vi "HGCalSensorTestingPanel.vi"() -> ()   [LabVIEW 2015]
uses:
  <vilib>/Utility/file.llb/Write Delimited Spreadsheet (string).vi
panel:
  out "XY Graph 2":cluster{"Y":dbl[], "Y":dbl[]}[](graph)
  out "return count 5":u32
  in  "write buffer 2":string
  out "return count 4":u32
  in  "VISA QT7600":refnum<visa-resource-name>
  in  "write buffer":string
  out "VISA out 3":refnum<visa-resource-name>
  out "return count 3":u32
  in  "byte count 2":u32
  out "XY Graph":cluster{"Y":dbl[], "Y":dbl[]}[](graph)
  out "VISA out 2":refnum<visa-resource-name>
  out "return count 2":u32
  out "error out 2":errorcluster
  in  "byte count":u32
  in  "HP":refnum<visa-resource-name>
  out "VISA out":refnum<visa-resource-name>
  out "return count":u32
  in  "error in":errorcluster
  in  "Switch":refnum<visa-resource-name>
  in  "Measurement Data":string[][](table)
  in  "OK Button":bool
  in  "Delay (s):":dbl
  in  "Channel:":dbl
  in  "Voltage (V):":dbl
  out "Channel:":dbl format="%#3_6g"
  out "mV(nA)":dbl
  out "pF":dbl
  out "V":dbl
  out "nA":dbl
  # "C"
  # "A"
  # "V"
  # "1M"
  # "1M"
  # "Single Measurement"
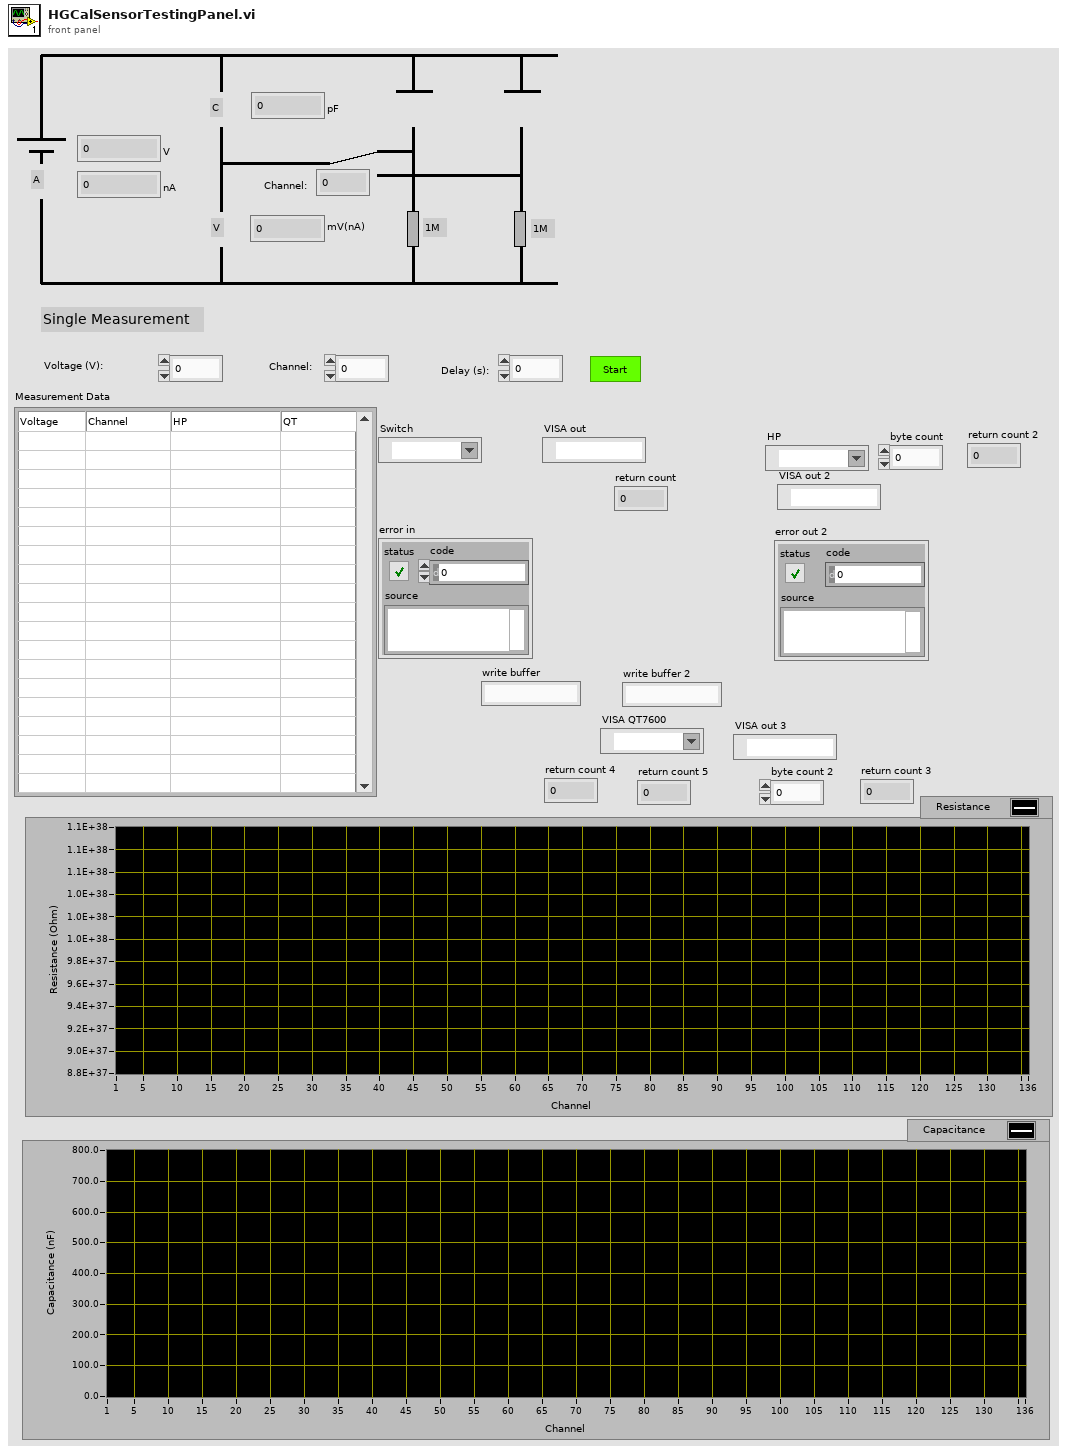
[diagram p1: front panel]
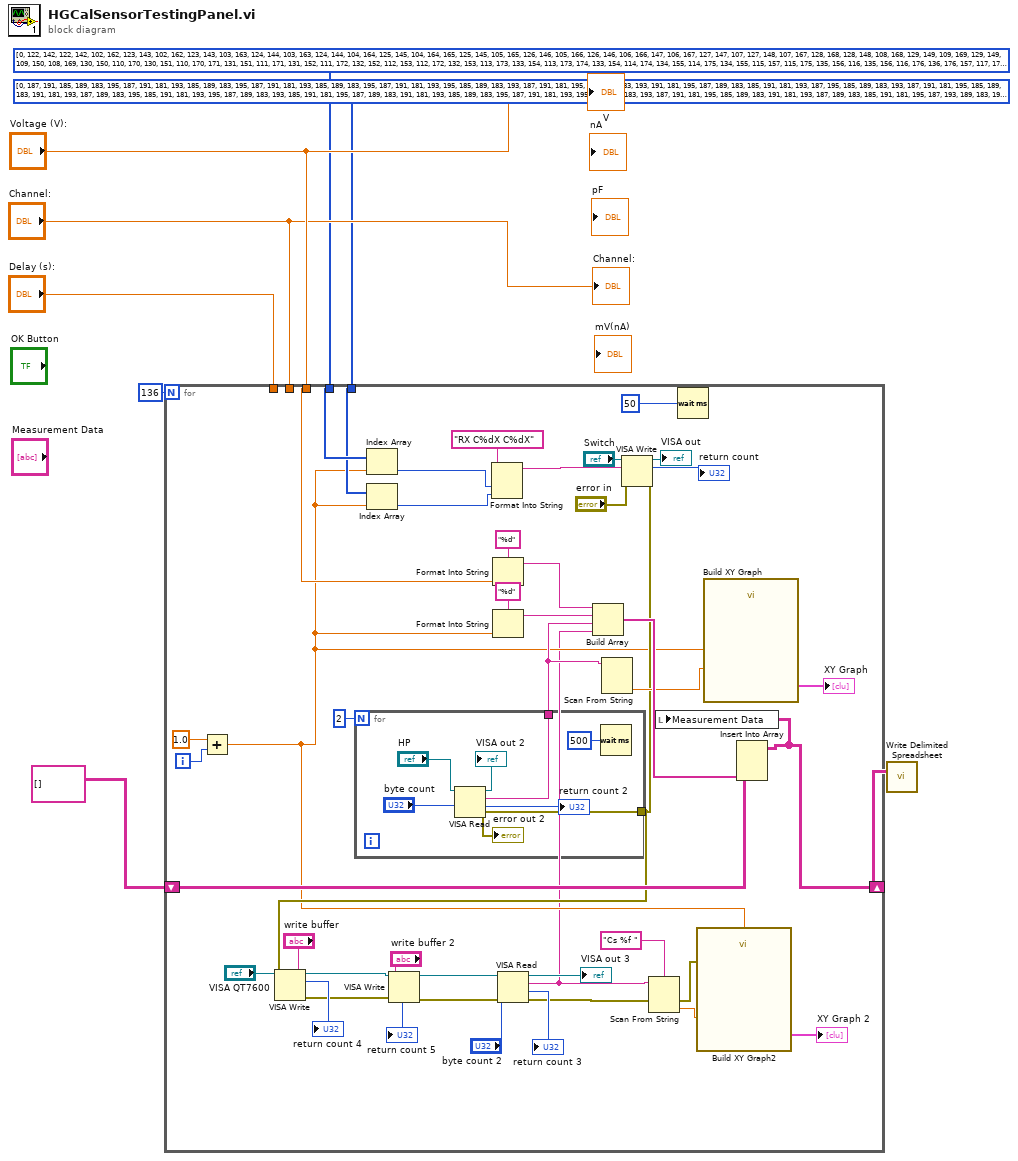
[diagram p0: block diagram]
diagram:
  n1 = for {
    N: 136 -> [_]
    shift-right: [w44] -> w3
    shift-left: string[][] [] -> [w53]
    tunnel: "Voltage (V):" -> [w52]
    tunnel: "Channel:" -> [_]
    tunnel: "Delay (s):" -> [_]
    tunnel: i32[] [0, 122, 142, 122, 142, 102, 162, 123, 143, 102, 162, 123, 143, 103, 163, 124, 144, 103, 163, 124, 144, 104, 164, 125, 145, 104, 164, 165, 125, 145, 105, 165, 126, 146, 105, 166, 126, 146, 106, 166, 147, 106, 167, 127, 147, 107, 127, 148, 107, 167, 128, 168, 128, 148, 108, 168, 129, 149, 109, 169, 129, 149, 109, 150, 108, 169, 130, 150, 110, 170, 130, 151, 110, 170, 171, 131, 151, 111, 171, 131, 152, 111, 172, 132, 152, 112, 153, 112, 172, 132, 153, 113, 173, 133, 154, 113, 173, 174, 133, 154, 114, 174, 134, 155, 114, 175, 134, 155, 115, 157, 115, 175, 135, 156, 116, 135, 156, 116, 176, 136, 176, 157, 117, 177, 136, 158, 117, 177, 137, 137, 158, 118, 178, 138, 138, 159, 178] -> [w43]
    tunnel: i32[] [0, 187, 191, 185, 189, 183, 195, 187, 191, 181, 193, 185, 189, 183, 195, 187, 191, 181, 193, 185, 189, 183, 195, 187, 191, 181, 193, 195, 185, 189, 183, 193, 187, 191, 181, 195, 185, 189, 183, 193, 191, 181, 195, 187, 189, 183, 185, 191, 181, 193, 187, 195, 185, 189, 183, 193, 187, 191, 181, 195, 185, 189, 183, 191, 181, 193, 187, 189, 183, 195, 185, 191, 181, 193, 195, 187, 189, 183, 193, 185, 191, 181, 195, 187, 189, 183, 191, 181, 193, 185, 189, 183, 195, 187, 191, 181, 193, 195, 185, 189, 183, 193, 187, 191, 181, 195, 185, 189, 183, 191, 181, 193, 187, 189, 183, 185, 191, 181, 195, 187, 193, 189, 183, 195, 185, 191, 181, 193, 187, 185, 189, 183, 195, 187, 185, 191, 193] -> [w42]
    i -> [w46]
    n2 = Add(x=1.0, y=w46) -> (x+y=w14:dbl)
    n3 = Index Array(array=w43, index=w14) -> (element=w41:i32)
    n4 = Index Array(array=w42, index=w14) -> (element=w40:i32)
    n5 = Format Into String(format string="RX C%dX C%dX", w41, w40) -> (resulting string=w35:string)  [unwired: 2 in, 1 out]
    n6 = Format Into String(format string="%d", w52) -> (resulting string=w51:string)  [unwired: 2 in, 1 out]
    n7 = Format Into String(format string="%d", w14) -> (resulting string=w33:string)  [unwired: 2 in, 1 out]
    n8 = VISA Write(VISA resource name="Switch", write buffer=w35, error in (no error)="error in") -> (VISA resource name out=→"VISA out":refnum<visa-resource-name>, return count=→"return count":u32, error out=w16:errorcluster)
    n9 = VISA Write(VISA resource name="VISA QT7600", write buffer="write buffer", error in (no error)=w16) -> (VISA resource name out=w18:refnum<visa-resource-name>, return count=→"return count 4":u32, error out=w20:errorcluster)
    n10 = for {
      N: 2 -> [_]
      tunnel: [w56] -> w29
      tunnel: w16 -> [w54]
      n11 = VISA Read(VISA resource name="HP", byte count="byte count", error in (no error)=w54) -> (VISA resource name out=→"VISA out 2":refnum<visa-resource-name>, read buffer=w56:string, return count=→"return count 2":u32, error out=→"error out 2":errorcluster)
      n12 = Wait (ms)(milliseconds to wait=u32 500) -> ()  [unwired: 1 out]
    }
    n13 = VISA Write(VISA resource name=w18, write buffer="write buffer 2", error in (no error)=w20) -> (VISA resource name out=w17:refnum<visa-resource-name>, return count=→"return count 5":u32, error out=w19:errorcluster)
    n14 = VISA Read(VISA resource name=w17, byte count="byte count 2", error in (no error)=w19) -> (VISA resource name out=→"VISA out 3":refnum<visa-resource-name>, read buffer=w12:string, return count=→"return count 3":u32, error out=w11:errorcluster)
    n15 = Build Array(w51, w33, w29, w12) -> (w50:string[])
    n16 = Scan From String(input string=w29) -> (output 1=w30:dbl)  [unwired: 4 in, 3 out]
    n17 = Scan From String(format string="Cs %f ", input string=w12, error in=w11) -> (error out=w10:errorcluster, output 1=w13:dbl)  [unwired: 2 in, 2 out]
    n18 = Wait (ms)(milliseconds to wait=u32 50 ("millisecond timer value")) -> ()  [unwired: 1 out]
    n19 = call "Build XY Graph2"("error in (no error)"=w10, "Y Input"=w13, "X Input"=w14) -> ("XY Graph"=→"XY Graph 2":cluster{"X":dbl[], "Y":dbl[]}[])  [unwired: 7 in, 1 out]
    n20 = call "Build XY Graph"("Y Input"=w30, "X Input"=w14) -> ("XY Graph"=→"XY Graph":cluster{"X":dbl[], "Y":dbl[]}[])  [unwired: 8 in, 1 out]
    n21 = Insert Into Array(array=w53, new element=w50) -> (w44:string[][])  [unwired: 2 in]
    n22 = local write "Measurement Data"(w44) -> ()
  }
  n23 = call-poly <vilib>:"Write Delimited Spreadsheet.vi"("2D data"=w3) -> ()  [unwired: 13 in, 2 out]
  "V" <- "Voltage (V):"
  "Channel:" <- "Channel:"
